vi "TSPopup.Register.vi"(4 "Col (unwired = all columns)":i32=-2, 6 "Row (unwired = all rows)":i32=-2, 7 "Tag (none)":string, 8 "error in (no error)":errorcluster, 9 "Parameters":T1={"Prop Type"=enum."String", "Initial Value"=variant, "Caption Strings"=[], "Ring Strings"=[], "Cell Rect"={"left"=0, "top"=0, "right"=0, "bottom"=0}, "Mouse Coords"={"x"=0, "y"=0}, "Call Data"=variant}, 11 "Ctl Refnum":refnum<vi>) -> (0 "error out":errorcluster, 3 "dup ref out":refnum<vi>)   [LabVIEW 2013]
doc: "Register a control location with some associated Popup Parameters. These will be retrieved by using the \"TSPopup.Lookup.vi\" in a <Mouse Down?> event. \n\nRegistration can be done for an exact cell, a column, a row, or an entire control. Retrieval of parameters will be done by searching in that order.\n\n<B>Ctl Refnum</B> - Refnum of control that is being registered (allowed control types : String, Table, Listbox, Multicolumn Listbox, Tree)\n<B>Popup Parameters</B> - Parameters for showing the Type Sensitive Popup.\n<B>Tag</B> - For tree controls, this is the row's tag. Unwired or blank equals all rows.\n<B>Row</B> - Row being registered. Unwired or (< -1) equals all rows.\n<B>Col</B> - Column being registered. Unwired or (< -1) equals all rows.\n\nType Sensitive Popup \nCopyright © 2007, J. David Saunders\nAll rights reserved."
uses:
  TSPopup.Popup Call Parameters.ctl
  TSPopup.Data Type.ctl
  Private/TSPopup.Popup Operation.ctl
panel:
  # "Type Sensitive Popup \nCopyright © 2007, J. David Saunders\nAll rights reserved."
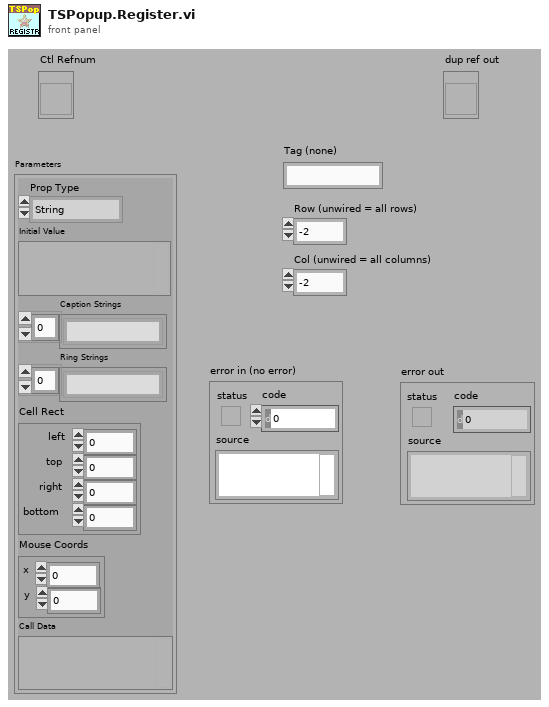
[diagram p1: front panel]
types:
  T1 = typedef "TSPopup.Popup Call Parameters.ctl" = cluster{"Prop Type":T2, "Initial Value":variant, "Caption Strings":string[], "Ring Strings":string[], "Cell Rect":cluster{"left":i16, "top":i16, "right":i16, "bottom":i16}, "Mouse Coords":cluster{"x":i16, "y":i16}, "Call Data":variant}
  T2 = typedef "TSPopup.Data Type.ctl" = enum16{"Unkown", "NO POPUP", "String", "Integer", "Float", "Color", "Boolean", "Ring", "Captioned String", "Captioned Integer", "Button Color", "2 Int Cluster", "4 Int Cluster"}
  T3 = typedef "TSPopup.Popup Operation.ctl" = enum16{"Show", "Initialize", "Close", "Popup Done", "Register a Location's Type", "Retrieve Location's Type"}
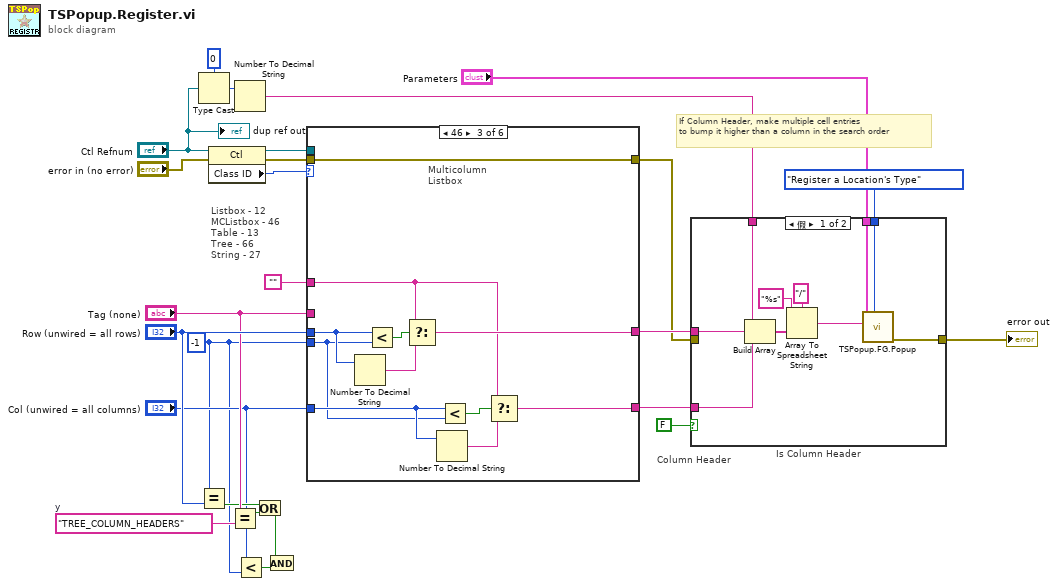
[diagram p0: block diagram]
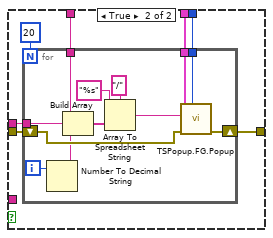
[diagram p2: hidden frame]
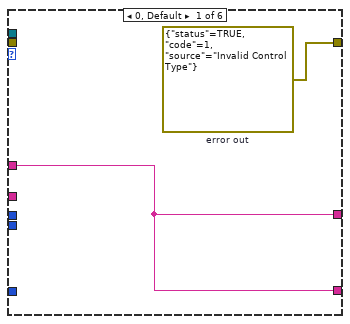
[diagram p3: hidden frame]
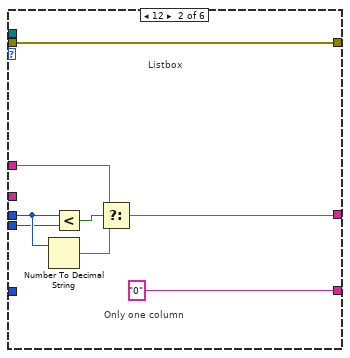
[diagram p4: hidden frame]
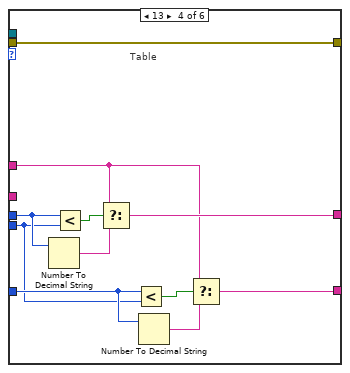
[diagram p5: hidden frame]
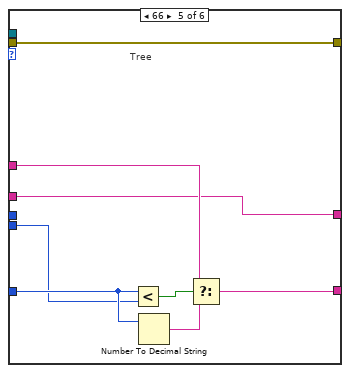
[diagram p6: hidden frame]
diagram:
  w12 = "TREE_COLUMN_HEADERS"  # y
  w4 = -1 ("y")
  # "If Column Header, make multiple cell entries\nto bump it higher than a column in the search order"
  # "Column Header"
  # "Listbox - 12\nMCListbox - 46\nTable - 13\nTree - 66\nString - 27"
  n1 = Type Cast(type=0, x="Ctl Refnum") -> (*(type *) &x=w22:i32)
  n2 = Equal?(x=w4, y="Row (unwired = all rows)") -> (x = y?=w10:bool)
  n3 = property class="Ctl"(reference="Ctl Refnum", error in="error in (no error)") -> (reference out=w24:refnum<vi>, error out=w16:errorcluster, "Class ID"=w25:u32)
  n4 = Equal?(x="Tag (none)", y=w12) -> (x = y?=w11:bool)
  n5 = Number To Decimal String(number=w22) -> (decimal integer string=w21:string)  [unwired: 1 in]
  n6 = Less?(x="Col (unwired = all columns)", y=w4) -> (x < y?=w3:bool)
  n7 = Or(x=w10, y=w11) -> (x .or. y?=w2:bool)
  n8 = And(x=w2, y=w3) -> ()  [unwired: 1 out]
  n9 = case shown="46" w25 {
    tunnel: w24 -> [_ _ _ _ _ _]
    tunnel: "Tag (none)" -> [_ _ _ _ w62 _]
    tunnel: "Row (unwired = all rows)" -> [_ w30 w39 w51 _ _]
    tunnel: "Col (unwired = all columns)" -> [_ _ w38 w49 w60 _]
    tunnel: "" -> [w27 w34 w42 w53 w63 w67]
    tunnel: [w27 w33 w45 w56 w62 w67] -> w19
    tunnel: [w27 "0" w43 w54 w64 w67] -> w18
    tunnel: w16 -> [_ w31 w41 w52 w61 w66]
    tunnel: [w26 w31 w41 w52 w61 w66] -> w6
    tunnel: w4 -> [_ w29 w36 w48 w59 _]
    frame 0, Default {
      w26 = errorcluster {"status"=TRUE, "code"=1, "source"="Invalid Control Type"}  # error out
    }
    frame 12 {
      # "Only one column"
      # "Listbox"
      n10 = Number To Decimal String(number=w30) -> (decimal integer string=w35:string)  [unwired: 1 in]
      n11 = Less?(x=w30, y=w29) -> (x < y?=w28:bool)
      n12 = Select(t=w34, s=w28, f=w35) -> (s? t:f=w33:string)
    }
    frame 46 {
      # "Multicolumn\nListbox"
      n13 = Number To Decimal String(number=w39) -> (decimal integer string=w46:string)  [unwired: 1 in]
      n14 = Less?(x=w39, y=w36) -> (x < y?=w40:bool)
      n15 = Select(t=w42, s=w40, f=w46) -> (s? t:f=w45:string)
      n16 = Number To Decimal String(number=w38) -> (decimal integer string=w44:string)  [unwired: 1 in]
      n17 = Less?(x=w38, y=w36) -> (x < y?=w37:bool)
      n18 = Select(t=w42, s=w37, f=w44) -> (s? t:f=w43:string)
    }
    frame 13 {
      # "Table"
      n19 = Number To Decimal String(number=w51) -> (decimal integer string=w57:string)  [unwired: 1 in]
      n20 = Less?(x=w51, y=w48) -> (x < y?=w50:bool)
      n21 = Select(t=w53, s=w50, f=w57) -> (s? t:f=w56:string)
      n22 = Less?(x=w49, y=w48) -> (x < y?=w47:bool)
      n23 = Number To Decimal String(number=w49) -> (decimal integer string=w55:string)  [unwired: 1 in]
      n24 = Select(t=w53, s=w47, f=w55) -> (s? t:f=w54:string)
    }
    frame 66 {
      # "Tree"
      n25 = Less?(x=w60, y=w59) -> (x < y?=w58:bool)
      n26 = Number To Decimal String(number=w60) -> (decimal integer string=w65:string)  [unwired: 1 in]
      n27 = Select(t=w63, s=w58, f=w65) -> (s? t:f=w64:string)
    }
    frame 27 {
      # "String"
    }
  }
  n28 = case "Is Column Header" shown="假" FALSE {
    tunnel: w21 -> [w74 w84]
    tunnel: w19 -> [w73 w83]
    tunnel: w18 -> [w72 _]
    tunnel: [w70 w82] -> w9
    tunnel: "Parameters" -> [w69 w80]
    tunnel: TSPopup.Popup_Operation."Register a Location's Type" ("Popup Operation") -> [w68 w81]
    tunnel: w6 -> [_ w79]
    frame False {
      n29 = Build Array(w74, w73, w72) -> (w77:string[])
      n30 = Array To Spreadsheet String(delimiter (Tab)="/", array=w77, 3:"%s" ("format string")) -> (spreadsheet string=w71:string)
      n31 = call "TSPopup.FG.Popup.vi"("Popup Operation"=w68, "Encoded Location"=w71, "Popup Parameters"=w69) -> ("error out"=w70:errorcluster)  [unwired: 5 in, 3 out]
    }
    frame True {
      n32 = for {
        N: 20 -> [_]
        tunnel: w84 -> [w93]
        tunnel: w83 -> [w92]
        tunnel: w81 -> [w89]
        tunnel: w80 -> [w88]
        shift-right: [w90] -> w82
        shift-left: w79 -> [w87]
        i -> [w86]
        n33 = Number To Decimal String(number=w86) -> (decimal integer string=w85:string)  [unwired: 1 in]
        n34 = Build Array(w93, w92, w85) -> (w96:string[])
        n35 = Array To Spreadsheet String(delimiter (Tab)="/", array=w96, 3:"%s" ("format string")) -> (spreadsheet string=w91:string)
        n36 = call "TSPopup.FG.Popup.vi"("Popup Operation"=w89, "error in (no error)"=w87, "Encoded Location"=w91, "Popup Parameters"=w88) -> ("error out"=w90:errorcluster)  [unwired: 4 in, 3 out]
      }
    }
  }
  "error out" <- w9
  "dup ref out" <- "Ctl Refnum"
